vi "Get Type.vi"(11 "DoublePanel in":refnum<class "DoublePanel.lvclass">) -> (2 "Type":refnum<class "Type.lvclass">)   [LabVIEW 2020, in "Conditum-Tools.lvlib" / "DoublePanel.lvclass"]
uses:
  DoublePanel.lvclass
  Conditum-Clone/Columns/Type/Type.lvclass
  DoublePanel.lvclass/DoublePanel.ctl
  Conditum-Clone/Columns/Double/Double.lvclass
  C:/dev/lv20CE/lv-conditum-tools/Conditum-Clone/Columns/Type/Type.lvclass
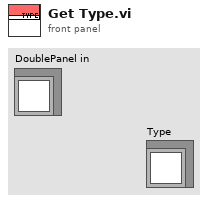
[diagram p1: front panel]
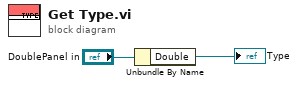
[diagram p0: block diagram]
diagram:
  n1 = Unbundle By Name("DoublePanel in") -> ("Double"=→"Type":refnum<class "Double.lvclass">)
